vi "AppendReplaceScript.vi"(7 "Replace":bool, 10 "New Script":string, 11 "Old Script":string) -> (3 "Result":string)   [LabVIEW 2021, in "ScriptManager.lvlib"]
uses:
  ScriptManager.lvlib
  <vilib>/regexp/Match Regular Expression.xnode
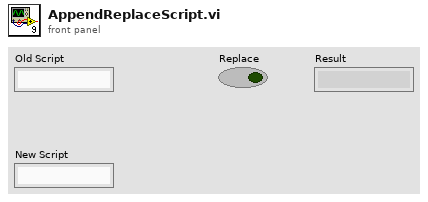
[diagram p1: front panel]
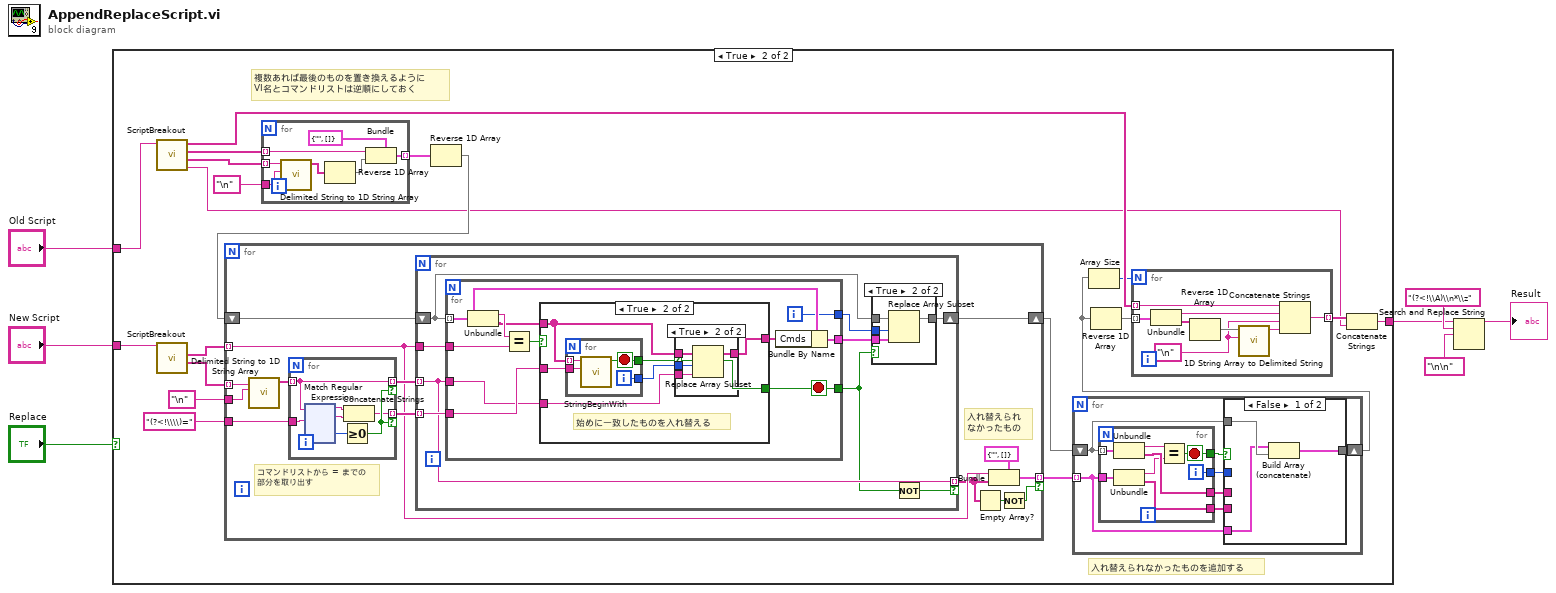
[diagram p0: block diagram]
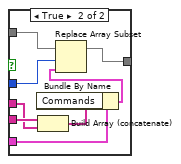
[diagram p3: hidden frame]
diagram:
  n1 = case shown="True" "Replace" {
    tunnel: "Old Script" -> [w8 w16]
    tunnel: "New Script" -> [_ w15]
    tunnel: [w8 w14] -> w2
    frame False {
    }
    frame True {
      # "入れ替えられなかったものを追加する"
      # "複数あれば最後のものを置き換えるように\nVI名とコマンドリストは逆順にしておく"
      n2 = call "ScriptBreakout.vi"("Script"=w16) -> ("Rest"=w13:string, "Commands"=w25:string[], "VI Name"=w26:string[], "Padding"=w18:string[])  [unwired: 7 in]
      n3 = call "ScriptBreakout.vi"("Script"=w15) -> ("Commands"=w27:string[], "VI Name"=w28:string[])  [unwired: 7 in, 2 out]
      n4 = for {
        tunnel: w26 -> [w60] mode=indexing
        tunnel: w25 -> [w61] mode=indexing
        tunnel: "\n" ("delimiter") -> [w57]
        tunnel: [w56] -> w23 mode=indexing
        n5 = call <vilib>:"Delimited String to 1D String Array.vi"("delimiter"=w57, "delimited string"=w61) -> ("string array"=w59:string[])  [unwired: 9 in]
        n6 = Reverse 1D Array(array=w59) -> (reversed array=w58:string[])
        n7 = Bundle(cluster=cluster{"VI":string, "Cmds":string[]} {"VI"="", "Cmds"=[]}, "VI"=w60, "Cmds"=w58) -> (w56:cluster{"VI":string, "Cmds":string[]})
      }
      n8 = Reverse 1D Array(array=w23) -> (reversed array=w22:cluster{"VI":string, "Cmds":string[]}[])
      n9 = for {
        tunnel: w27 -> [w75] mode=indexing
        tunnel: w28 -> [w66] mode=indexing
        tunnel: "\n" ("delimiter") -> [w70]
        tunnel: "(?<!\\\\)=" ("delimiter") -> [w69]
        shift-right: [w68] -> w11
        shift-left: w22 -> [w72]
        tunnel: [w65] -> w12 mode=indexing if=w62
        # "入れ替えられ\nなかったもの"
        # "コマンドリストから = までの\n部分を取り出す"
        n10 = call <vilib>:"Delimited String to 1D String Array.vi"("delimiter"=w70, "delimited string"=w75) -> ("string array"=w74:string[])  [unwired: 9 in]
        n11 = for {
          tunnel: [w80] -> w73 mode=indexing if=w81
          tunnel: [w77] -> w71 mode=indexing if=w81
          tunnel: w74 -> [w77] mode=indexing
          tunnel: w69 -> [w78]
          n12 = xnode "Match Regular Expression"("input string"=w77, "regular expression"=w78) -> ("before match"=w82:string, "whole match"=w79:string, "offset past match"=w76:i32)  [unwired: 4 in, 2 out]
          n13 = Greater Or Equal To 0?(x=w76) -> (x >= 0?=w81:bool)
          n14 = Concatenate Strings(w82, w79) -> (w80:string)
        }
        n15 = for {
          tunnel: w73 -> [w207] mode=indexing
          tunnel: w66 -> [w208]
          tunnel: w71 -> [w206] mode=indexing
          shift-right: [w204] -> w68
          shift-left: w72 -> [w203]
          tunnel: [w206] -> w64 mode=indexing if=w205
          n16 = for {
            tunnel: w203 -> [w218] mode=indexing
            tunnel: w208 -> [w224]
            tunnel: w207 -> [w220]
            tunnel: w206 -> [w219]
            tunnel: [w216] -> w202
            tunnel: [w215] -> w200
            tunnel: [w214] -> w201
            i -> [w214]
            stop <- w215 stop-if-true
            n17 = Unbundle(w218) -> ("VI"=w222:string, "Cmds"=w221:string[])
            n18 = Equal?(x=w222, y=w224) -> (x = y?=w223:bool)
            n19 = case shown="True" w223 {
              tunnel: w221 -> [w225 w228]
              tunnel: w220 -> [_ w231]
              tunnel: w219 -> [_ w229]
              tunnel: [w225 w226] -> w217
              tunnel: [_ w227] -> w215
              frame False {
              }
              frame True {
                # "始めに一致したものを入れ替える"
                n20 = for {
                  tunnel: w228 -> [w239] mode=indexing
                  tunnel: w231 -> [w240]
                  tunnel: [w238] -> w227
                  tunnel: [w237] -> w230
                  i -> [w237]
                  stop <- w238 stop-if-true
                  n21 = call "StringBeginWith.vi"("Begin With"=w240, "String"=w239) -> ("StringBeginWith"=w238:bool)  [unwired: 9 in]
                }
                n22 = case shown="True" w227 {
                  tunnel: w230 -> [_ w236]
                  tunnel: w229 -> [_ w235]
                  tunnel: w228 -> [w232 w234]
                  tunnel: [w232 w233] -> w226
                  frame False {
                  }
                  frame True {
                    n23 = Replace Array Subset(array=w234, new element=w235, index=w236) -> (w233:string[])
                  }
                }
              }
            }
            n24 = Bundle By Name(cluster=w218, "Cmds"=w217) -> (w216:cluster{"VI":string, "Cmds":string[]})
          }
          n25 = case shown="True" w200 {
            tunnel: [w209 w213] -> w204
            tunnel: w203 -> [w209 w212]
            tunnel: w202 -> [_ w211]
            tunnel: w201 -> [_ w210]
            frame False {
            }
            frame True {
              n26 = Replace Array Subset(array=w212, new element=w211, index=w210) -> (w213:cluster{"VI":string, "Cmds":string[]}[])
            }
          }
          n27 = Not(x=w200) -> (.not. x?=w205:bool)
        }
        n28 = Empty Array?(array=w64) -> (empty?=w63:bool)
        n29 = Bundle(cluster=cluster{"VI":string, "Commands":string[]} {"VI"="", "Commands"=[]}, "VI"=w66, "Commands"=w64) -> (w65:cluster{"VI":string, "Commands":string[]})
        n30 = Not(x=w63) -> (.not. x?=w62:bool)
      }
      n31 = for {
        tunnel: w12 -> [w30] mode=indexing
        shift-right: [w29] -> w9
        shift-left: w11 -> [w32]
        n32 = for {
          tunnel: w32 -> [w50] mode=indexing
          tunnel: w30 -> [w54]
          tunnel: [w52] -> w35
          tunnel: [w51] -> w34
          tunnel: [w49] -> w33
          tunnel: [w47] -> w31
          i -> [w51]
          stop <- w52 stop-if-true
          n33 = Unbundle(w50) -> ("VI"=w53:string, "Cmds"=w49:string[])
          n34 = Unbundle(w54) -> ("VI"=w48:string, "Commands"=w47:string[])
          n35 = Equal?(x=w53, y=w48) -> (x = y?=w52:bool)
        }
        n36 = case shown="False" w35 {
          tunnel: w34 -> [_ w45]
          tunnel: w33 -> [_ w43]
          tunnel: w32 -> [w38 w46]
          tunnel: w31 -> [_ w44]
          tunnel: w30 -> [w37 w42]
          tunnel: [w36 w39] -> w29
          frame False {
            n37 = Build Array (concatenate)(w37, w38) -> (w36:cluster{"VI":string, "Cmds":string[]}[])
          }
          frame True {
            n38 = Build Array (concatenate)(w44, w43) -> (w41:string[])
            n39 = Bundle By Name(cluster=w42, "Commands"=w41) -> (w40:cluster{"VI":string, "Commands":string[]})
            n40 = Replace Array Subset(array=w46, new element=w40, index=w45) -> (w39:cluster{"VI":string, "Cmds":string[]}[])
          }
        }
      }
      n41 = Array Size(array=w9) -> (size(s)=w10:i32)
      n42 = Reverse 1D Array(array=w9) -> (reversed array=w19:cluster{"VI":string, "Cmds":string[]}[])
      n43 = for {
        N: w10 -> [_]
        tunnel: w19 -> [w248] mode=indexing
        tunnel: w18 -> [w242] mode=indexing
        tunnel: [w241] -> w17 mode=indexing
        w243 = "\n" ("delimiter")
        n44 = Unbundle(w248) -> ("VI"=w244:string, "Cmds"=w247:string[])
        n45 = Reverse 1D Array(array=w247) -> (reversed array=w246:string[])
        n46 = call <vilib>:"1D String Array to Delimited String.vi"("delimiter"=w243, "string array"=w246) -> ("delimited string"=w245:string)  [unwired: 9 in]
        n47 = Concatenate Strings(w242, w244, w243, w245) -> (w241:string)
      }
      n48 = Concatenate Strings(w17, w13) -> (w14:string)
    }
  }
  n49 = Search and Replace String(input string=w2, search string="(?<!\\A)\\n*\\z", replace string="\n\n" ("replace string (\"\")")) -> (result string=→"Result":string)  [unwired: 5 in, 3 out]
